vi "serialize-xml-variant-attributes.vi"() -> ()   [LabVIEW 2020]
uses:
  classes/MsgSerializer.XML/MsgSerializer.XML.lvclass
  C:/projects/caraya/src/classes/MsgSerializer/MsgSerializer.lvclass
  classes/MsgSerializer.XML/format -- enum.ctl
  classes/MsgSerializer.XML/decimal-notation -- enum.ctl
  classes/MsgSerializer.XML/MsgSerializer.XML.lvclass/MsgSerializer.XML.ctl
  classes/MsgSerializer/MsgSerializer.lvclass/MsgSerializer.ctl
  classes/Properties.Test/Properties.Test.lvclass
  C:/projects/caraya/src/classes/Properties/Properties.lvclass
  classes/Properties.Assert/Properties.Assert.lvclass
  <vilib>/regexp/Match Regular Expression.xnode
  classes/Test/Test.lvclass
  classes/MsgSerializer/MsgSerializer.lvclass
  classes/Assert/Assert.lvclass
  classes/Properties/Properties.lvclass
panel:
  out "Serialized Test Case":string
  out "Serialized Test Suite":string
  out "Serialized Cluster":string
  out "Serialized Variant Attributes":string
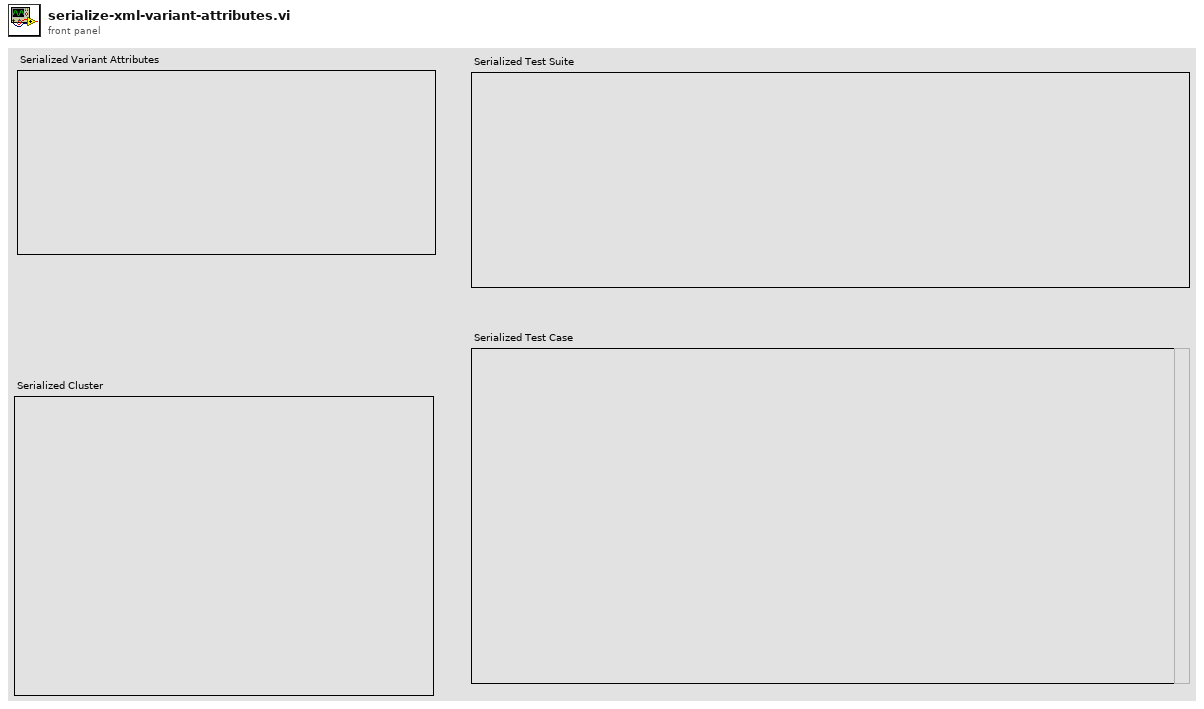
[diagram p1: front panel]
types:
  T1 = typedef "Caraya.lvlib/MsgSerializer.lvclass/decimal-notation -- enum.ctl" = enum16{"System-defined", "dot-notation", "comma-notation"}
  T2 = typedef "Caraya.lvlib/MsgSerializer.XML.lvclass/format -- enum.ctl" = enum16{"value", "tag", "property"}
  T3 = cluster{"classname":string, "name":string, "time":dbl, "skipped":bool, "failure":bool, "failure message":string, "failure description":string, "properties":variant, "measurements":variant, "limits":variant}[]
  T4 = cluster{"name":string, "errors":u32, "skipped":u32, "tests":u32, "failures":u32, "time":dbl, "timestamp":timestamp, "Call Chain":string[], "properties":variant}
  T5 = cluster{"status":bool, "code":i32, "inner":cluster{"status":bool, "code":i32, "timestamp":timestamp, "properties":variant}, "class":refnum<class "MsgSerializer.XML.lvclass">}
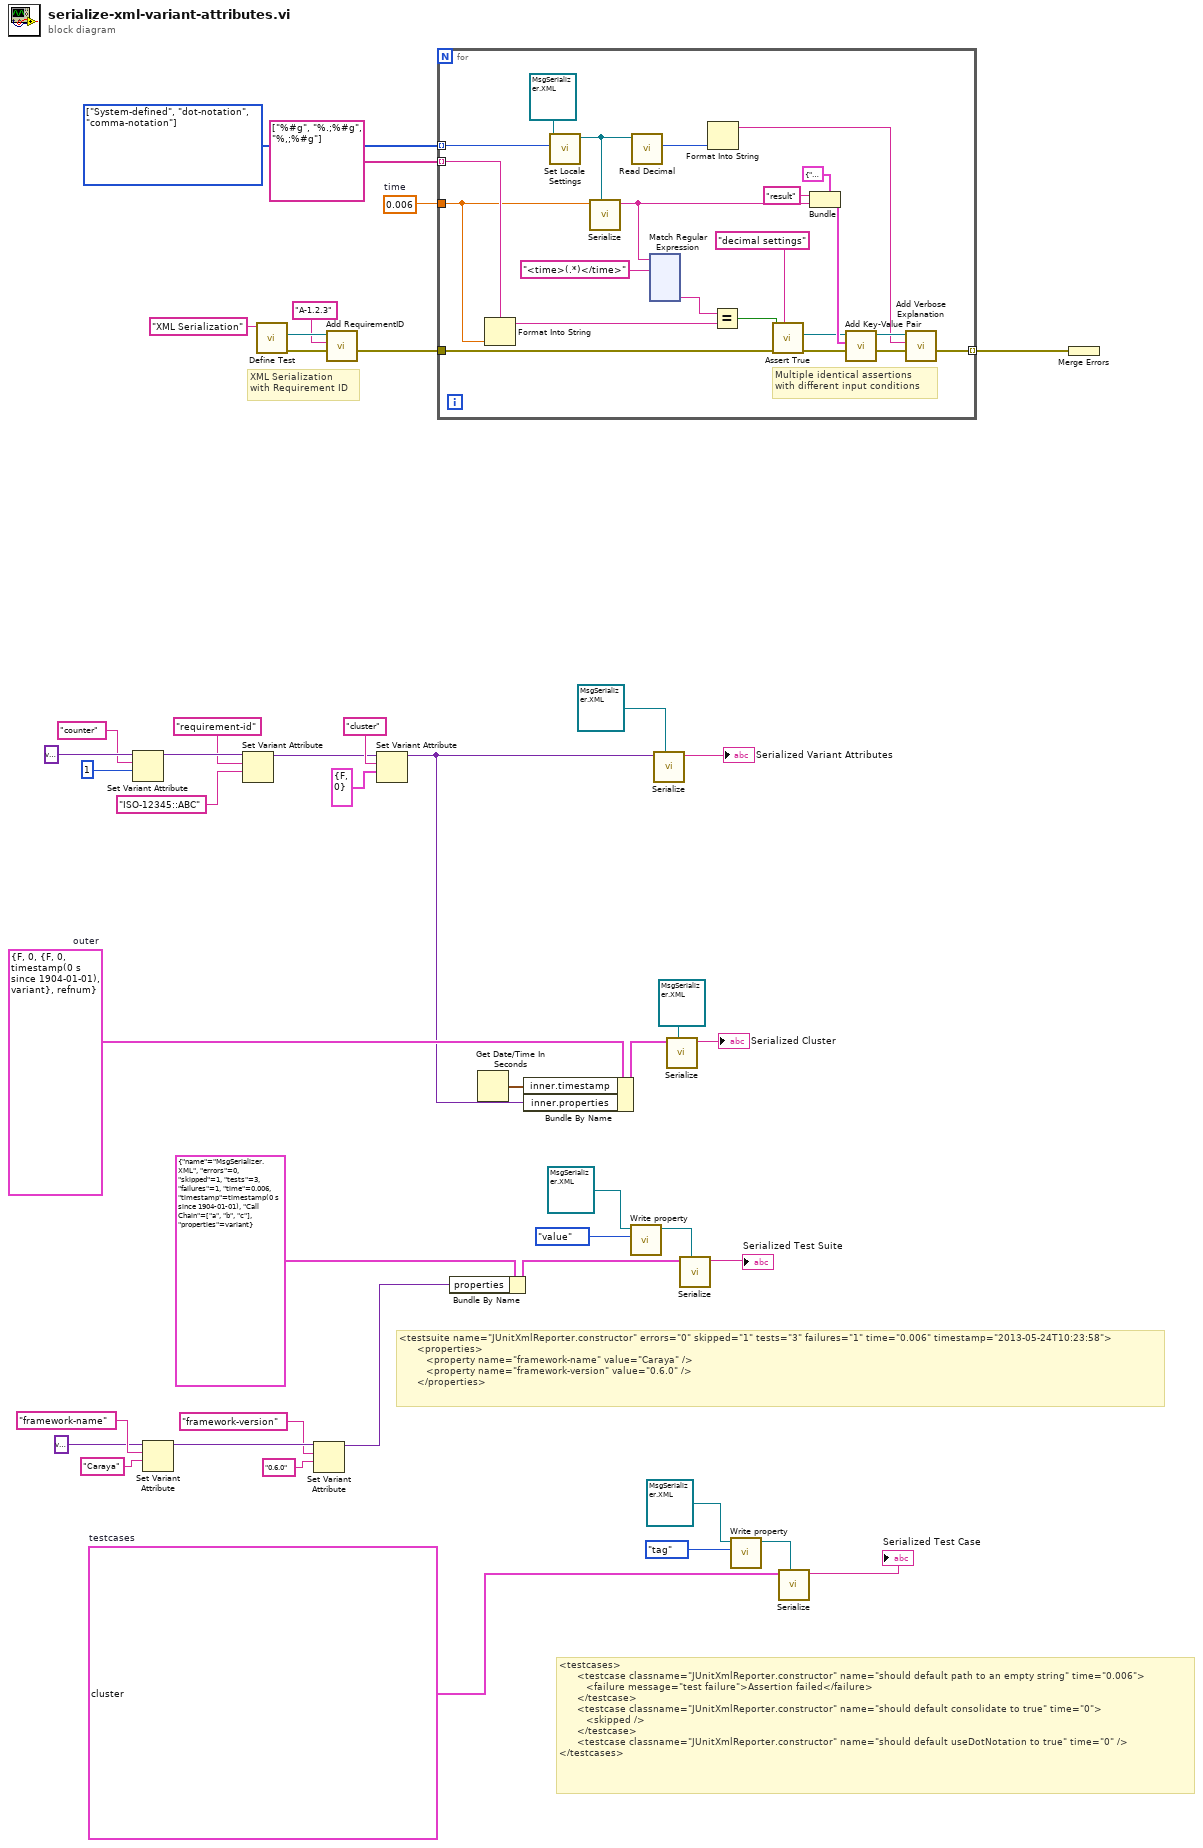
[diagram p0: block diagram]
diagram:
  w5 = 0.006  # time
  w8 = T1[] [enum."System-defined", enum."dot-notation", enum."comma-notation"] items=["System-defined", "dot-notation", "comma-notation"]
  w13 = T3 [{"classname"="MsgSerializer.XML", "name"="should default path to an empty string", "time"=0.006, "skipped"=FALSE, "failure"=TRUE, "failure message"="test failure", "failure description"="", "properties"=variant, "measurements"=variant, "limits"=variant}, {"classname"="MsgSerializer.XML", "name"="should default useDotNotation to true", "time"=0.0, "skipped"=FALSE, "failure"=FALSE, "failure message"="", "failure description"="", "properties"=variant, "measurements"=variant, "limits"=variant}, {"classname"="MsgSerializer.XML", "name"="should default consolidate to true", "time"=0.0, "skipped"=FALSE, "failure"=FALSE, "failure message"="", "failure description"="", "properties"=variant, "measurements"=variant, "limits"=variant}]  # testcases
  w32 = T5 {"status"=FALSE, "code"=0, "inner"={"status"=FALSE, "code"=0, "timestamp"=timestamp(0 s since 1904-01-01), "properties"=variant}, "class"=refnum}  # outer
  # "XML Serialization\nwith Requirement ID"
  # "<testcases>\n      <testcase classname=\"JUnitXmlReporter.constructor\" name=\"should default path to an empty string\" time=\"0.006\">\n         <failure message=\"test failure\">Assertion failed</failure>\n      </testcase>\n      <testcase classname=\"JUnitXmlReporter.constructor\" name=\"should default consolidate to true\" time=\"0\">\n         <skipped />\n      </testcase>\n      <testcase classname=\"JUnitXmlReporter.constructor\" name=\"should default useDotNotation to true\" time=\"0\" />\n</testcases>"
  # "<testsuite name=\"JUnitXmlReporter.constructor\" errors=\"0\" skipped=\"1\" tests=\"3\" failures=\"1\" time=\"0.006\" timestamp=\"2013-05-24T10:23:58\">\n      <properties>\n         <property name=\"framework-name\" value=\"Caraya\" />\n         <property name=\"framework-version\" value=\"0.6.0\" />\n      </properties>"
  n1 = Set Variant Attribute(Variant=variant ("variant"), name="counter", value=1) -> (Variant out=w42:variant)  [unwired: 1 in, 2 out]
  n2 = Set Variant Attribute(Variant=variant ("variant"), name="framework-name", value="Caraya" ("name")) -> (Variant out=w24:variant)  [unwired: 1 in, 2 out]
  n3 = Set Variant Attribute(Variant=w42, name="requirement-id", value="ISO-12345::ABC" ("name")) -> (Variant out=w30:variant)  [unwired: 1 in, 2 out]
  n4 = call "Define Test.vi"("Label (VI Title)"="XML Serialization") -> ("error out"=w3:errorcluster, "Properties.Test"=w4:refnum<class "Properties.Test.lvclass">)  [unwired: 9 in]
  n5 = Set Variant Attribute(Variant=w24, name="framework-version", value="0.6.0" ("name")) -> (Variant out=w22:variant)  [unwired: 1 in, 2 out]
  n6 = call "Add RequirementID.vi"("error in (no error)"=w3, "Requirement ID"="A-1.2.3" ("Label (VI Title)"), "Properties"=w4) -> ("error out"=w1:errorcluster)  [unwired: 7 in, 1 out]
  n7 = Set Variant Attribute(Variant=w30, name="cluster", value=cluster{"status":bool, "code":i32} {"status"=FALSE, "code"=0} ("error constant")) -> (Variant out=w11:variant)  [unwired: 1 in, 2 out]
  n8 = for {
    tunnel: w8 -> [w48] mode=indexing
    tunnel: string[] ["%#g", "%.;%#g", "%,;%#g"] -> [w63] mode=indexing
    tunnel: w1 -> [w61]
    tunnel: [w52] -> w6 mode=indexing
    tunnel: w5 -> [w56]
    # "Multiple identical assertions\nwith different input conditions"
    n9 = Format Into String(format string=w63, w56) -> (resulting string=w64:string)  [unwired: 2 in, 1 out]
    n10 = call "Set Locale Settings.vi"("Decimal"=w48, "MsgSerializer"=refnum<class "MsgSerializer.XML.lvclass"> refnum ("Caraya.lvlib:MsgSerializer.XMLProperty.lvclass")) -> ("MsgSerializer"=w49:refnum<class "MsgSerializer.XML.lvclass">)  [unwired: 9 in]
    n11 = call-dynamic "Serialize.vi"("MsgSerializer"=w49, "Value"=w56) -> ("Serialized Message"=w46:string)  [unwired: 8 in, 1 out]
    n12 = call "Read Decimal.vi"("MsgSerializer"=w49) -> ("Decimal"=w47:T1)  [unwired: 9 in, 1 out]
    n13 = xnode "Match Regular Expression"("input string"=w46, "regular expression"="<time>(.*)</time>") -> ("submatch 1"=w65:string)  [unwired: 4 in, 5 out]
    n14 = Format Into String(w47) -> (resulting string=w50:string)  [unwired: 3 in, 1 out]
    n15 = Equal?(x=w65, y=w64) -> (x = y?=w45:bool)
    n16 = call "Assert True.vi"("Label"="decimal settings" ("format string"), "error in (no error)"=w61, "True?"=w45) -> ("error out"=w55:errorcluster, "Properties"=w54:refnum<class "Properties.Assert.lvclass">)  [unwired: 7 in]
    n17 = Bundle(cluster=cluster{"key":string, "value":variant} {"key"="", "value"=variant} ("entry"), "key"="result", "value"=w46) -> (w58:cluster{"key":string, "value":variant})
    n18 = call "Add Key-Value Pair.vi"("error in (no error)"=w55, "entry"=w58, "Properties in"=w54) -> ("error out"=w53:errorcluster, "Properties out"=w51:refnum<class "Properties.Assert.lvclass">)  [unwired: 7 in]
    n19 = call "Add Verbose Explanation.vi"("error in (no error)"=w53, "Verbose Explanation"=w50, "Properties"=w51) -> ("error out"=w52:errorcluster)  [unwired: 7 in, 1 out]
  }
  n20 = Bundle By Name(cluster=T4 {"name"="MsgSerializer.XML", "errors"=0, "skipped"=1, "tests"=3, "failures"=1, "time"=0.006, "timestamp"=timestamp(0 s since 1904-01-01), "Call Chain"=["a", "b", "c"], "properties"=variant} ("testsuite"), "properties"=w22) -> (w20:T4)
  n21 = Get Date/Time In Seconds() -> (seconds since 1Jan1904=w33:timestamp)
  n22 = Bundle By Name(cluster=w32, "inner.timestamp"=w33, "inner.properties"=w11) -> (w31:T5)
  n23 = call "Write property.vi"("format"=format_--_enum."value", "MsgSerializer.XMLProperty in"=refnum<class "MsgSerializer.XML.lvclass"> refnum ("Caraya.lvlib:MsgSerializer.XMLProperty.lvclass")) -> ("MsgSerializer.XMLProperty out"=w17:refnum<class "MsgSerializer.XML.lvclass">)  [unwired: 9 in]
  n24 = call-dynamic "Serialize.vi"("MsgSerializer"=refnum<class "MsgSerializer.XML.lvclass"> refnum ("Caraya.lvlib:MsgSerializer.XMLProperty.lvclass"), "Value"=w11) -> ("Serialized Message"=→"Serialized Variant Attributes":string)  [unwired: 8 in, 1 out]
  n25 = call-dynamic "Serialize.vi"("MsgSerializer"=refnum<class "MsgSerializer.XML.lvclass"> refnum ("Caraya.lvlib:MsgSerializer.XMLProperty.lvclass"), "Value"=w31) -> ("Serialized Message"=→"Serialized Cluster":string)  [unwired: 8 in, 1 out]
  n26 = call-dynamic "Serialize.vi"("MsgSerializer"=w17, "Value"=w20) -> ("Serialized Message"=→"Serialized Test Suite":string)  [unwired: 8 in, 1 out]
  n27 = call "Write property.vi"("format"=format_--_enum."tag", "MsgSerializer.XMLProperty in"=refnum<class "MsgSerializer.XML.lvclass"> refnum ("Caraya.lvlib:MsgSerializer.XMLProperty.lvclass")) -> ("MsgSerializer.XMLProperty out"=w16:refnum<class "MsgSerializer.XML.lvclass">)  [unwired: 9 in]
  n28 = call-dynamic "Serialize.vi"("MsgSerializer"=w16, "Value"=w13) -> ("Serialized Message"=→"Serialized Test Case":string)  [unwired: 8 in, 1 out]
  n29 = Merge Errors(w6) -> ()  [unwired: 1 out]
